vi "Get Info.vi"(8 "error in (no error)":errorcluster, 11 "NI SMU in":refnum<class "NI SMU.lvclass">) -> (0 "error out":errorcluster, 2 "Info":variant, 3 "NI SMU out":refnum<class "NI SMU.lvclass">)   [LabVIEW 2020, in "NI SMU.lvlib" / "NI SMU.lvclass"]
uses:
  NI SMU.lvclass
  NI SMU.lvclass/NI SMU.ctl
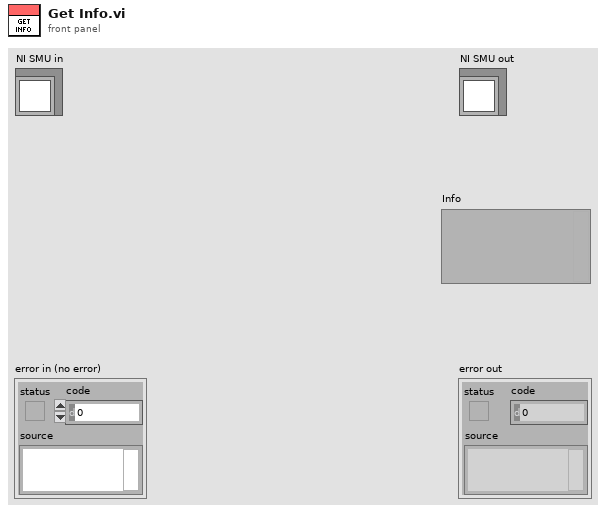
[diagram p1: front panel]
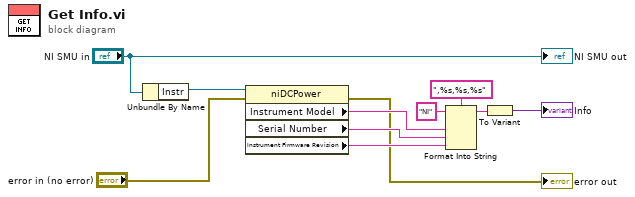
[diagram p0: block diagram]
diagram:
  n1 = Unbundle By Name("NI SMU in") -> ("Instr"=w2:refnum<k15>)
  n2 = property class="niDCPower"(reference=w2, error in="error in (no error)") -> (error out=→"error out":errorcluster, "Instrument Model"=w7:string, "Serial Number"=w9:string, "Instrument Firmware Revision"=w8:string)  [unwired: 1 out]
  n3 = Format Into String(format string=",%s,%s,%s", initial string="NI", w7, w9, w8) -> (resulting string=w10:string)  [unwired: 1 in, 1 out]
  n4 = To Variant(anything=w10) -> (Variant=→"Info":variant)
  "NI SMU out" <- "NI SMU in"
